vi "XIPIN_HDMI_1.4_2.0_Receiver_Subsystem_1_0.vi"   [LabVIEW 2017]
doc: "HDMI Receiver Subsystem supporting HDMI 1.4 and 2.0\n------------------------------------\n<b>Need License</b> : No"
uses:
  <vilib>/rvi/XilinxIP/XIPIN_XNode/niFpgaXIPIN.xnode
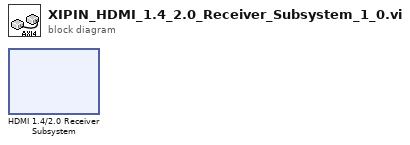
[diagram p0: block diagram]
diagram:
  n1 = xnode ("HDMI 1.4/2.0 Receiver Subsystem")() -> ()
